vi "getSensorData.vi"(2 "API-key":string, 6 "station id":u32=4551) -> (0 "value":T1, 5 "not-found":bool)   [LabVIEW 2024]
uses:
  <vilib>/httpClient/LabVIEWHTTPClient.lvlib
panel:
  out "Numeric":i32
  out "headers":string
  out "body":string
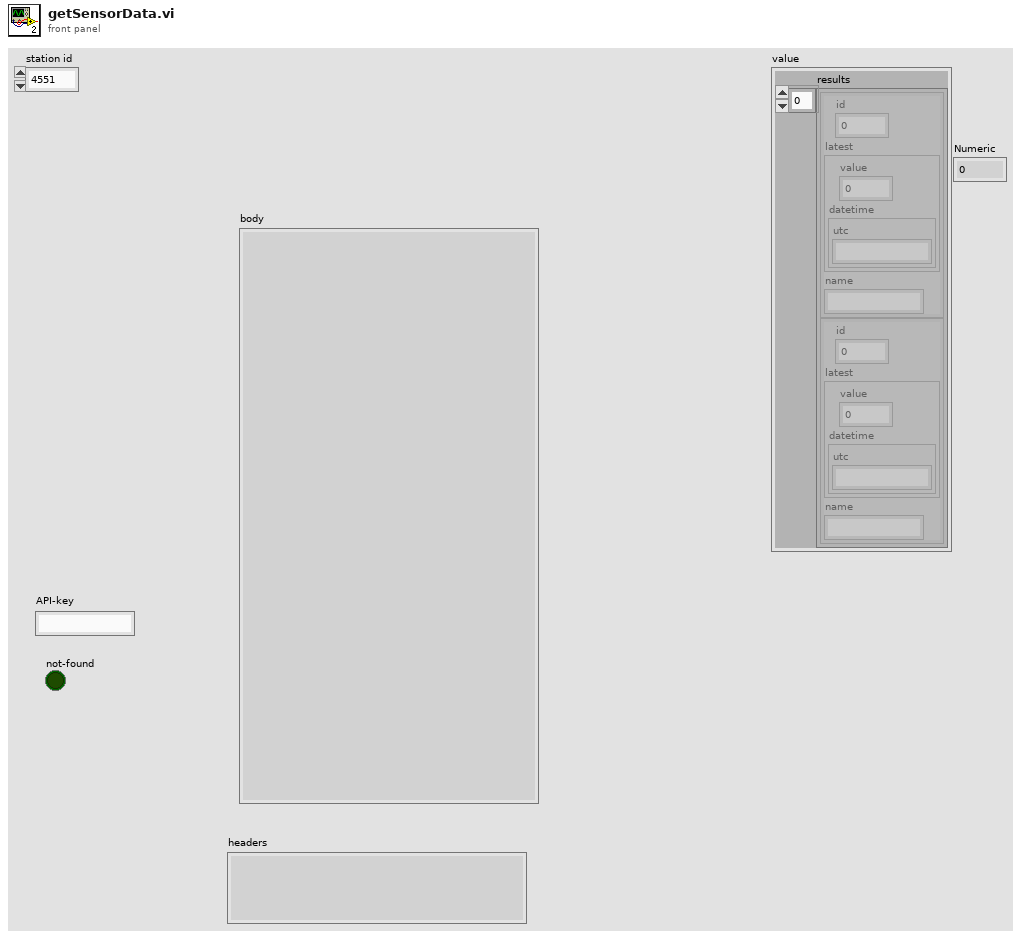
[diagram p1: front panel]
types:
  T1 = cluster{"results":cluster{"id":u16, "latest":cluster{"value":dbl, "datetime":cluster{"utc":string}}, "name":string}[]}
  T2 = typedef "LabVIEWHTTPClient.lvlib/ClientHandle.ctl" = refnum<k1>
  T3 = cluster{"results":cluster{"id":u32, "latest":cluster{"value":dbl, "datetime":cluster{"utc":string}}, "name":string}[]}
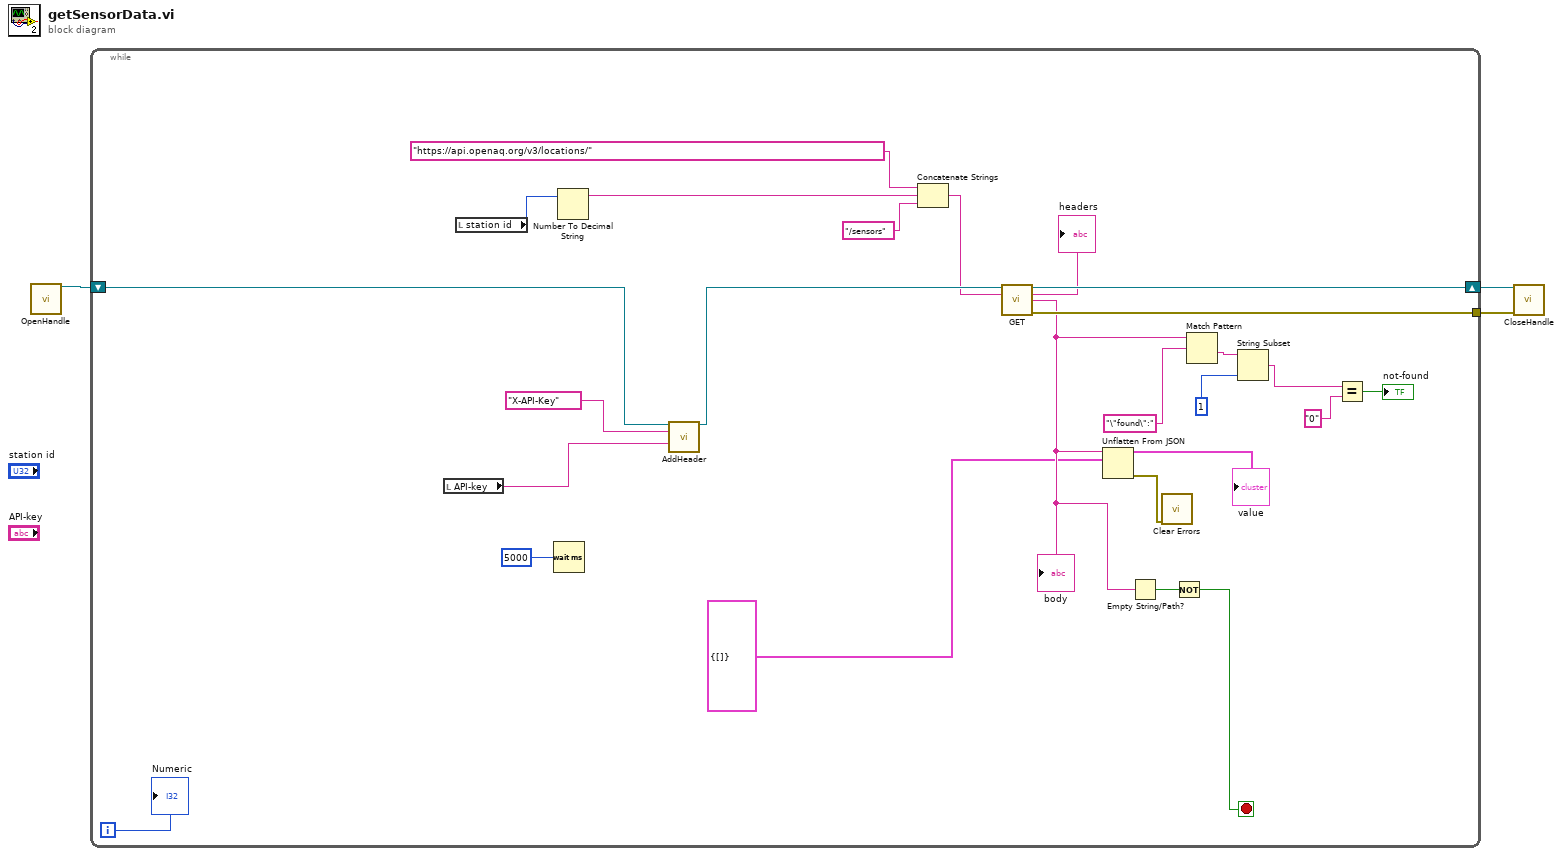
[diagram p0: block diagram]
diagram:
  n1 = call <vilib>:"OpenHandle.vi"() -> ("client handle out"=w1:T2)  [unwired: 14 in, 1 out]
  n2 = while {
    tunnel: [w28] -> w2
    shift-right: [w29] -> w3
    shift-left: w1 -> [w23]
    i -> [w4]
    stop <- w11 stop-if-true
    n3 = local read "API-key"() -> (w22:string)
    n4 = local read "station id"() -> (w6:u32)
    n5 = Wait (ms)(milliseconds to wait=u32 5000) -> ()  [unwired: 1 out]
    n6 = Number To Decimal String(number=w6) -> (decimal integer string=w8:string)  [unwired: 1 in]
    n7 = call <vilib>:"AddHeader.vi"("client handle"=w23, "header"="X-API-Key", "value"=w22) -> ("client handle out"=w26:T2)  [unwired: 11 in, 1 out]
    n8 = Concatenate Strings("https://api.openaq.org/v3/locations/", w8, "/sensors") -> (w5:string)
    n9 = call <vilib>:"GET.vi"("client handle"=w26, "url"=w5) -> ("client handle out"=w29:T2, "headers"=→"headers":string, "body"=w21:string, "error out"=w28:errorcluster)  [unwired: 10 in]
    "body" <- w21
    n10 = Unflatten From JSON(JSON string=w21, type and defaults=T3 {"results"=[]}) -> (value=→"value":T3, error out=w19:errorcluster)  [unwired: 5 in]
    n11 = Empty String/Path?(string/path=w21) -> (empty?=w20:bool)
    n12 = call <vilib>:"Clear Errors.vi"("error in (no error)"=w19) -> ()  [unwired: 5 in, 2 out]
    n13 = Not(x=w20) -> (.not. x?=w11:bool)
    n14 = Match Pattern(string=w21, regular expression="\"found\":") -> (after substring=w17:string)  [unwired: 1 in, 3 out]
    n15 = String Subset(string=w17, length (rest)=1 ("length (rest)")) -> (substring=w15:string)  [unwired: 1 in]
    n16 = Equal?(x=w15, y="0") -> (x = y?=→"not-found":bool)
    "Numeric" <- w4
  }
  n17 = call <vilib>:"CloseHandle.vi"("client handle"=w3, "error in (no error)"=w2) -> ()  [unwired: 13 in, 1 out]
